vi "ICA_16_Potluri - Copy.vi"() -> ()   [LabVIEW 2016]
uses:
  <vilib>/NXT/Block Support/NXT_OutputPort.ctl
  <vilib>/NXT/Dual Mode Library/Sensors/EV3_Color_Color.vi
  <vilib>/NXT/NXTIO Xnodes/NXTIONodeSubVIs/LEGOMoveAllMotors.vi
  <vilib>/NXT/Dual Mode Library/Waits/Wait_Num.vi
  <vilib>/NXT/NXTIO Xnodes/NXTIONodeSubVIs/NXTMotorRunDistance.vi
  <vilib>/NXT/NXTIO Xnodes/NXTIONodeSubVIs/LEGOStopAllMotors.vi
  <vilib>/NXT/Dual Mode Library/Sensors/EV3_Ultrasonic_CM.vi
  <vilib>/NXT/Subs/LVHSConnector.ctl
  <vilib>/NXT/NXTIO Xnodes/NXTIOXNode/NXTIO.xnode
  <vilib>/NXT/NXTIO Xnodes/AddressXNode/NXTIOAddress.xnode
  <vilib>/NXT/LegoClasses/BrickReference/BrickReference.lvclass
panel:
  out "Numeric":dbl
  out "Numeric 2":dbl
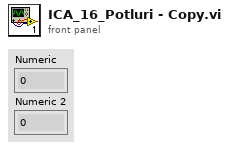
[diagram p1: front panel]
types:
  T1 = typedef "ColorSensorColors.ctl" = enum16{"No Color", "Black", "Blue", "Green", "Yellow", "Red", "White", "Brown"}
  T2 = typedef "LVHSConnector.ctl" = refnum<class "BrickReference.lvclass">
  T3 = typedef "NXT_OutputPort.ctl" = u8
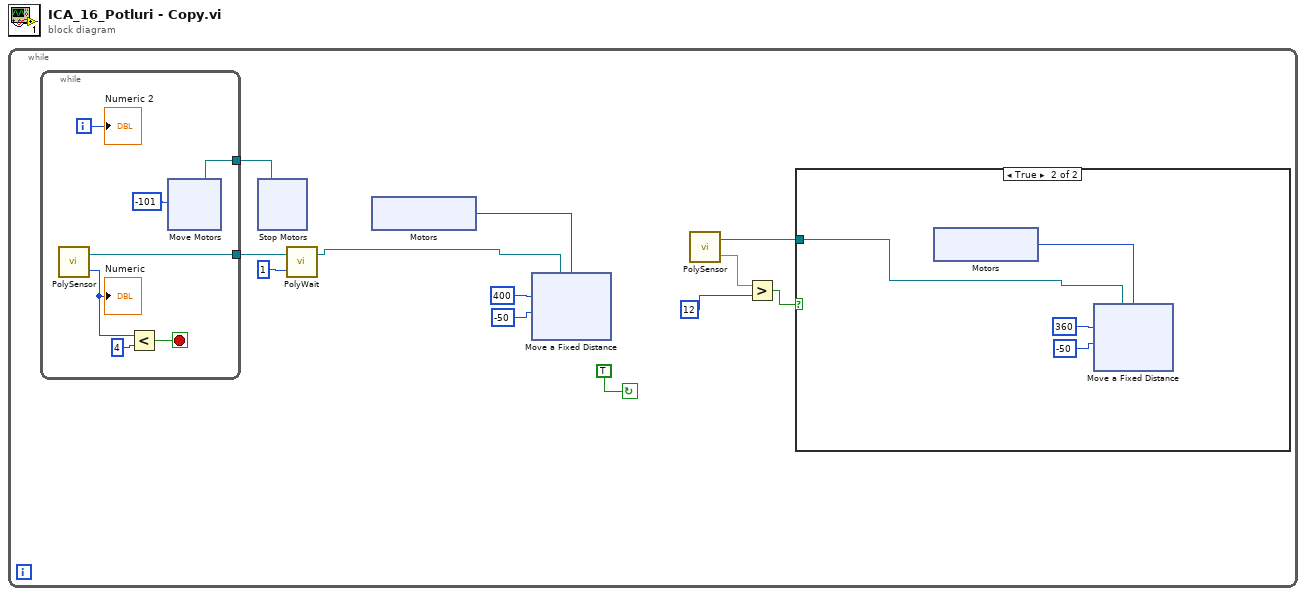
[diagram p0: block diagram]
diagram:
  n1 = while {
    stop <- TRUE continue-if-true
    n2 = while {
      tunnel: [w45] -> w9
      tunnel: [w44] -> w7
      i -> [w46]
      stop <- w49 stop-if-true
      n3 = call-poly <vilib>:"PolySensor.vi"() -> ("Detected Color"=w47:T1, "NXT/EV3"=w45:T2)  [unwired: 3 in]
      "Numeric" <- w47
      n4 = Less?(x=w47, y=4) -> (x < y?=w49:bool)
      n5 = xnode "Move Motors"("Power/Speed 1"=-101) -> ("NXT/EV3"=w44:T2)  [unwired: 2 in]
      "Numeric 2" <- w46
    }
    n6 = xnode "Stop Motors"("NXT/EV3"=w7) -> ()  [unwired: 1 in, 1 out]
    n7 = call-poly <vilib>:"PolyWait.vi"("Time (1 sec)"=1, "NXT/EV3"=w9) -> ("NXT/EV3"=w5:T2)  [unwired: 2 in]
    n8 = xnode "Motors"() -> ("Motor"=w10:T3)
    n9 = xnode "Move a Fixed Distance"("Speed 1"=-50, "Distance 1"=400, "Motors"=w10, "NXT/EV3"=w5) -> ()  [unwired: 1 out]
    n10 = call-poly <vilib>:"PolySensor.vi"() -> ("Centimeters"=w4:sgl, "NXT/EV3"=w1:T2)  [unwired: 3 in]
    n11 = Greater?(x=w4, y=12) -> (0:w2:bool)
    n12 = case shown="True" w2 {
      tunnel: w1 -> [_ w13]
      frame False {
      }
      frame True {
        n13 = xnode "Motors"() -> ("Motor"=w14:T3)
        n14 = xnode "Move a Fixed Distance"("Speed 1"=-50, "Distance 1"=360, "Motors"=w14, "NXT/EV3"=w13) -> ()  [unwired: 1 out]
      }
    }
  }
